vi "Read Firmware and Build Version.vi"(0 "Session Handle in":T1, 11 "error in (no error)":errorcluster) -> (4 "Session Handle out":T1, 6 "Build Date":string, 8 "Firmware Version":string, 15 "error out":errorcluster)   [LabVIEW 2015, in "PAS.lvclass"]
uses:
  PAS.lvclass
  Typedefs/Session Handle.ctl
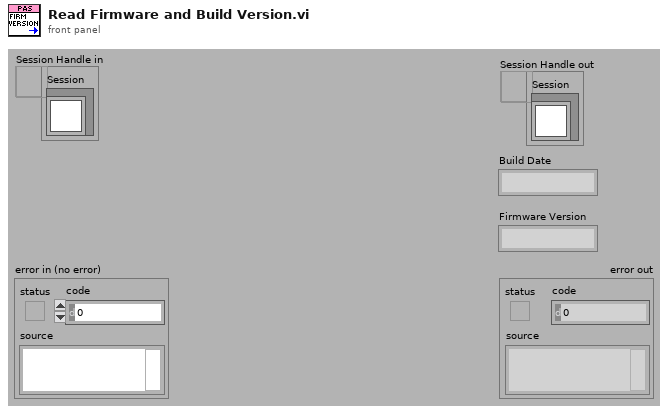
[diagram p1: front panel]
types:
  T1 = typedef "PAS.lvclass/Session Handle.ctl" = refnum<data-value>
  T2 = typedef "XNET Frame CAN.ctl" = cluster{"timestamp":timestamp, "payload":u8[], "identifier":u32, "type":T3, "extended?":bool, "echo?":bool}
  T3 = typedef "XNET Frame Type CAN.ctl" = u8
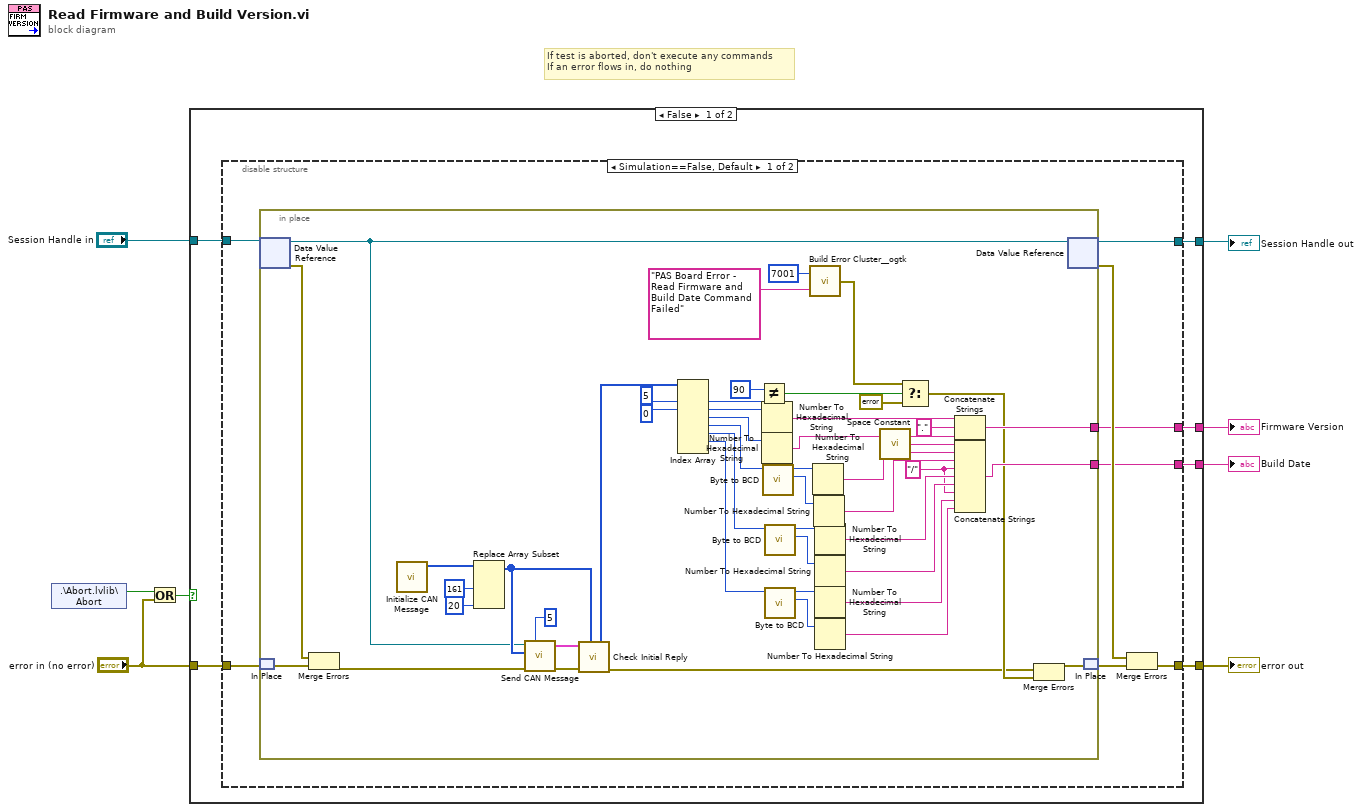
[diagram p0: block diagram]
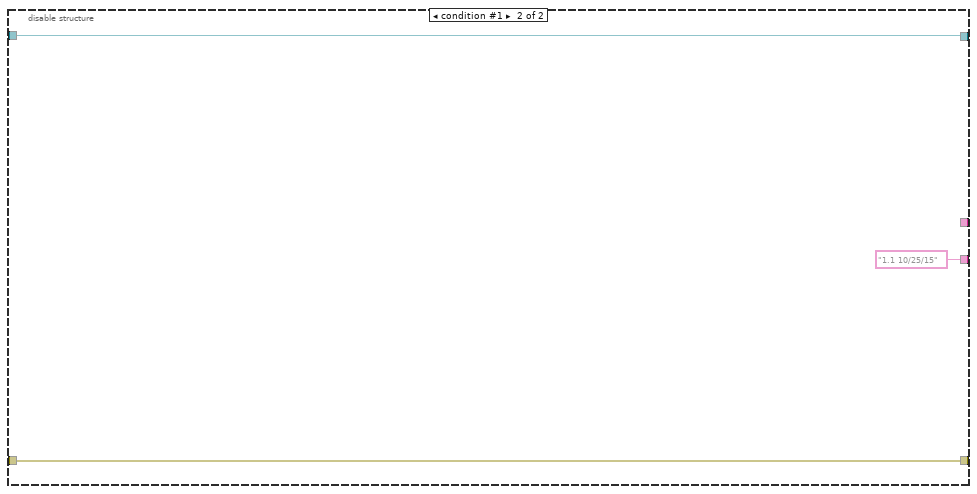
[diagram p2: hidden frame]
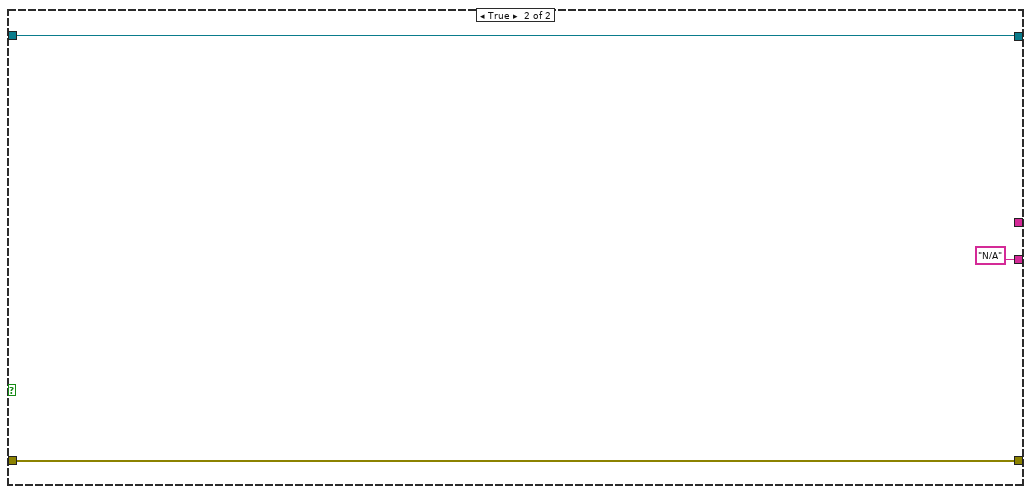
[diagram p3: hidden frame]
diagram:
  # "If test is aborted, don't execute any commands\nIf an error flows in, do nothing"
  n1 = shared-variable ".\\Abort.lvlib\\Abort"() -> (w5:bool)  [unwired: 1 in, 1 out]
  n2 = Or(x=w5, y="error in (no error)") -> (x .or. y?=w3:bool)
  n3 = case shown="False" w3 {
    tunnel: [w14 w76] -> w7
    tunnel: [w13 w75] -> w6
    tunnel: "Session Handle in" -> [w12 w76]
    tunnel: "error in (no error)" -> [w11 w75]
    tunnel: [w10 "N/A"] -> w2
    tunnel: [w9 _] -> w1
    frame False {
      n4 = disable-structure shown="Simulation==False, Default" {
        disable-tunnel: [w22 w73] -> w14
        disable-tunnel: [w19 w72] -> w13
        disable-tunnel: w12 -> [w18 w73]
        disable-tunnel: w11 -> [w17 w72]
        disable-tunnel: [w16 "1.1 10/25/15"] -> w10
        disable-tunnel: [w15 _] -> w9
        frame condition #0 (active) {
          n5 = in-place {
            in-place-border: [w30] -> w16
            in-place-border: [w26] -> w15
            w34 = "/" ("string")
            n6 = in-place-dvr #1(w18) -> (w61:refnum<class "PAS.lvclass">, w65:errorcluster)
            n7 = in-place-match #2(w17) -> (w64:errorcluster)
            n8 = Merge Errors(w65, w64) -> (w63:errorcluster)
            n9 = call "Initialize CAN Message.vi"() -> ("Initial Payload"=w67:u8[])  [unwired: 11 in]
            n10 = Replace Array Subset(array=w67, new element #1=u8 161 ("new element/subarray"), new element #2=u8 20 ("new element/subarray")) -> (w62:u8[])  [unwired: 2 in]
            n11 = call "Send CAN Message.vi"("Number of Retries"=5, "error in (no error)"=w63, "payload"=w62, "Gas In"=w61) -> ("error out"=w24:errorcluster, "Reply"=w59:T2[])  [unwired: 5 in, 1 out]
            n12 = call "Check Initial Reply.vi"("Write Message"=w62, "error in (no error)"=w24, "Reply"=w59) -> ("error out"=w23:errorcluster, "Data Packet"=w66:u8[])  [unwired: 5 in, 2 out]
            n13 = Index Array(array=w66, index #1=5 ("index"), index #2=0 ("index")) -> (element #1=w53:u8, element #2=w50:u8, element #3=w49:u8, element #4=w48:u8, element #5=w43:u8, element #6=w40:u8)  [unwired: 5 in, 1 out]
            n14 = Not Equal?(x=u8 90 ("new element/subarray"), y=w53) -> (x != y?=w51:bool)
            n15 = Number To Hexadecimal String(2:w50) -> (0:w27:string)  [unwired: 1 in]
            n16 = Number To Hexadecimal String(2:w49) -> (0:w28:string)  [unwired: 1 in]
            n17 = call "Byte to BCD.vi"("U8"=w48) -> ("low nibble"=w46:u8, "hi nibble"=w47:u8)  [unwired: 9 in]
            n18 = call "Byte to BCD.vi"("U8"=w43) -> ("low nibble"=w45:u8, "hi nibble"=w44:u8)  [unwired: 9 in]
            n19 = call "Byte to BCD.vi"("U8"=w40) -> ("low nibble"=w41:u8, "hi nibble"=w42:u8)  [unwired: 9 in]
            n20 = call <userlib>:"Build Error Cluster__ogtk.vi"("String to Prepend to source (\"\")"="PAS Board Error - Read Firmware and Build Date Command Failed" ("string"), "code"=7001) -> ("error out"=w56:errorcluster)
            n21 = Number To Hexadecimal String(2:w47) -> (0:w38:string)  [unwired: 1 in]
            n22 = Number To Hexadecimal String(2:w46) -> (0:w37:string)  [unwired: 1 in]
            n23 = Number To Hexadecimal String(2:w44) -> (0:w36:string)  [unwired: 1 in]
            n24 = Number To Hexadecimal String(2:w45) -> (0:w35:string)  [unwired: 1 in]
            n25 = Number To Hexadecimal String(2:w42) -> (0:w33:string)  [unwired: 1 in]
            n26 = Number To Hexadecimal String(2:w41) -> (0:w32:string)  [unwired: 1 in]
            n27 = call <vilib>:"Space Constant.vi"() -> ("String"=w31:string)
            n28 = Select(t=w56, s=w51, f=errorcluster {"status"=FALSE, "code"=0, "source"=""}) -> (s? t:f=w25:errorcluster)
            n29 = Concatenate Strings(w27, "." ("string"), w28) -> (w26:string)
            n30 = Concatenate Strings(w31, w38, w37, w34, w36, w35, w34, w33, w32) -> (w30:string)
            n31 = Merge Errors(w23, w25) -> (w68:errorcluster)
            n32 = in-place-dvr #1(w61) -> (w22:T1, w20:errorcluster)
            n33 = in-place-match #2(w68) -> (w21:errorcluster)
          }
          n34 = Merge Errors(w20, w21) -> (w19:errorcluster)
        }
        frame condition #1 {
        }
      }
    }
    frame True {
    }
  }
  "Session Handle out" <- w7
  "error out" <- w6
  "Build Date" <- w2
  "Firmware Version" <- w1
